vi "obsluga skal OY.vi"(8 "error in (no error)":errorcluster, 10 "PlotIdx":i32, 11 "WaveformGraph in":refnum<vi>) -> (0 "error out":errorcluster)   [LabVIEW 2014]
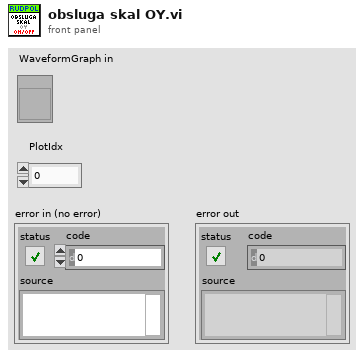
[diagram p1: front panel]
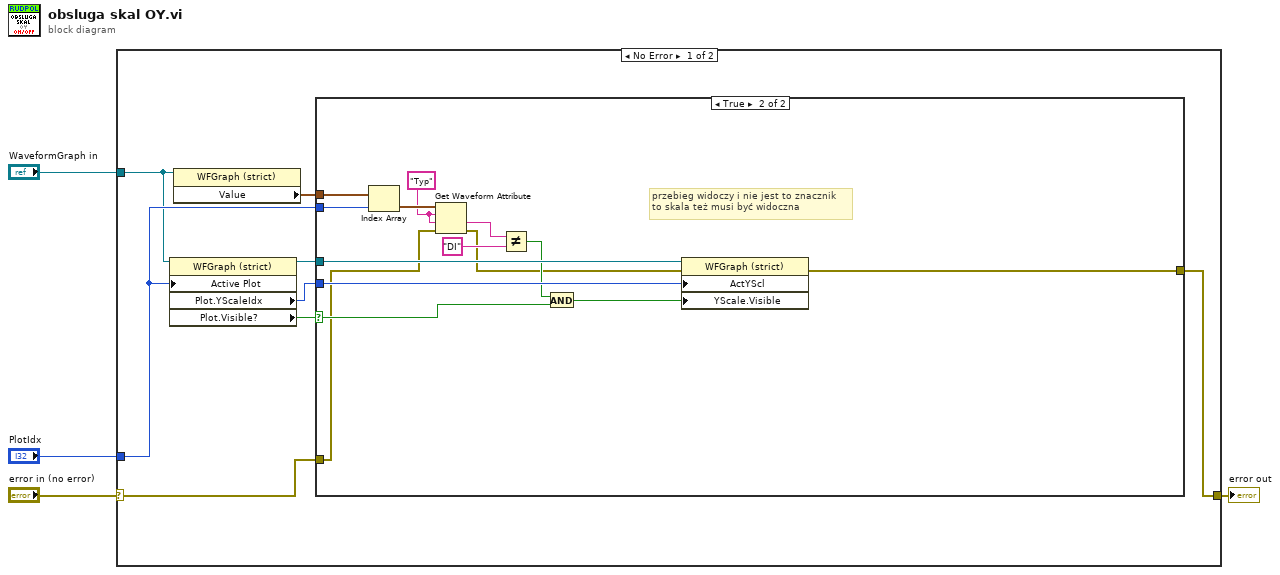
[diagram p0: block diagram]
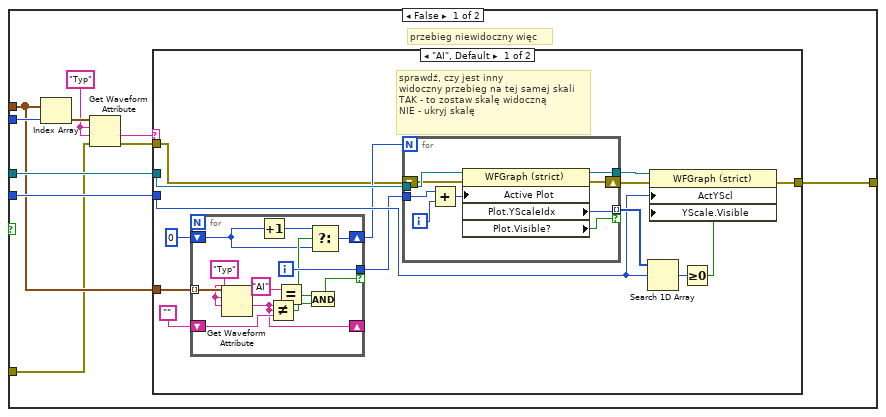
[diagram p2: hidden frame]
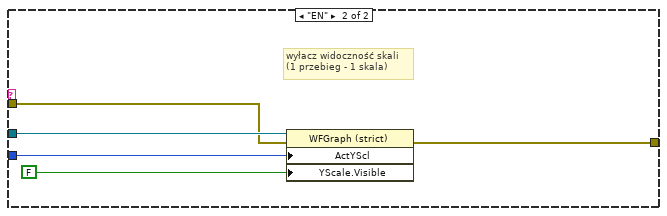
[diagram p3: hidden frame]
diagram:
  n1 = case shown="No Error" "error in (no error)" {
    selector: "error in (no error)" -> [w5 w77]
    tunnel: "PlotIdx" -> [w11 _]
    tunnel: "WaveformGraph in" -> [w10 _]
    tunnel: [w6 w77] -> w2
    frame No Error {
      n2 = property class="WFGraph (strict)"(reference=w10, "Active Plot"=w11) -> (reference out=w7:refnum<vi>, "Plot.YScaleIdx"=w8:u32, "Plot.Visible?"=w9:bool)  [unwired: 1 in, 1 out]
      n3 = property class="WFGraph (strict)"(reference=w10) -> ("Value"=w12:waveform(dbl)[])  [unwired: 1 in, 2 out]
      n4 = case shown="True" w9 {
        selector: w9 -> [_ w75]
        tunnel: w7 -> [w18 w76]
        tunnel: w8 -> [w17 w74]
        tunnel: w12 -> [w16 w71]
        tunnel: w11 -> [w22 w70]
        tunnel: w5 -> [w15 w64]
        tunnel: [w13 w72] -> w6
        frame False {
          w20 = "Typ"
          # "przebieg niewidoczny więc"
          n5 = Index Array(array=w16, index=w22) -> (element=w21:waveform(dbl))
          n6 = Get Waveform Attribute(4:w15, 5:w20, 6:w20, 7:w21) -> (0:w14:errorcluster, 1:w19:string)  [unwired: 2 out]
          n7 = case shown="\"AI\", Default" w19 {
            tunnel: w18 -> [w36 w62]
            tunnel: w17 -> [w32 w61]
            tunnel: w16 -> [w26 _]
            tunnel: w14 -> [w25 w58]
            tunnel: [w23 w59] -> w13
            frame "AI", Default {
              # "sprawdź, czy jest inny\nwidoczny przebieg na tej samej skali\nTAK - to zostaw skalę widoczną\nNIE - ukryj skalę"
              n8 = for {
                tunnel: w26 -> [w48] mode=indexing
                tunnel: [w46] -> w27 if=w42
                shift-right: [w41] -> _
                shift-left: "" -> [w45]
                shift-right: [w39] -> w28
                shift-left: 0 -> [w37]
                i -> [w46]
                w47 = "Typ"
                n9 = Get Waveform Attribute(5:w47, 6:w47, 7:w48) -> (1:w41:string)  [unwired: 1 in, 3 out]
                n10 = Increment(x=w37) -> (x+1=w38:i32)
                n11 = Not Equal?(x=w41, y=w45) -> (x != y?=w44:bool)
                n12 = Equal?(x="AI" ("y"), y=w41) -> (x = y?=w40:bool)
                n13 = And(x=w40, y=w44) -> (x .and. y?=w42:bool)
                n14 = Select(t=w38, s=w40, f=w37) -> (s? t:f=w39:i32)
              }
              n15 = for {
                N: w28 -> [_]
                tunnel: w36 -> [w57]
                tunnel: [w54] -> w35 mode=indexing if=w53
                tunnel: [w52] -> w33
                tunnel: w27 -> [w51]
                shift-right: [w49] -> w24
                shift-left: w25 -> [w50]
                i -> [w55]
                n16 = Add(x=w51, y=w55) -> (x+y=w56:i32)
                n17 = property class="WFGraph (strict)"(reference=w57, error in=w50, "Active Plot"=w56) -> (reference out=w52:refnum<vi>, error out=w49:errorcluster, "Plot.YScaleIdx"=w54:u32, "Plot.Visible?"=w53:bool)
              }
              n18 = Search 1D Array(1D array=w35, element=w32) -> (index of element=w34:i32)  [unwired: 1 in]
              n19 = Greater Or Equal To 0?(x=w34) -> (x >= 0?=w31:bool)
              n20 = property class="WFGraph (strict)"(reference=w33, error in=w24, "ActYScl"=w32, "YScale.Visible"=w31) -> (error out=w23:errorcluster)  [unwired: 1 out]
            }
            frame "EN" {
              # "wyłacz widoczność skali\n(1 przebieg - 1 skala)"
              n21 = property class="WFGraph (strict)"(reference=w62, error in=w58, "ActYScl"=w61, "YScale.Visible"=FALSE ("Y Scale.Visible")) -> (error out=w59:errorcluster)  [unwired: 1 out]
            }
          }
        }
        frame True {
          w68 = "Typ"
          # "przebieg widoczy i nie jest to znacznik\nto skala też musi być widoczna"
          n22 = Index Array(array=w71, index=w70) -> (element=w69:waveform(dbl))
          n23 = Get Waveform Attribute(4:w64, 5:w68, 6:w68, 7:w69) -> (0:w63:errorcluster, 1:w67:string)  [unwired: 2 out]
          n24 = Not Equal?(x=w67, y="DI") -> (x != y?=w65:bool)
          n25 = And(x=w65, y=w75) -> (x .and. y?=w73:bool)
          n26 = property class="WFGraph (strict)"(reference=w76, error in=w63, "ActYScl"=w74, "YScale.Visible"=w73) -> (error out=w72:errorcluster)  [unwired: 1 out]
        }
      }
    }
    frame Error {
    }
  }
  "error out" <- w2
